vi "Global Strings.vi"() -> ()   [LabVIEW 2024, in "Historical Table.lvlib" / "Historical Table.lvclass"]
uses:
  Historical Table.lvclass
panel:
  in  "Show":string="Show Table"
  in  "Update Period":string="Update period (s)"
  in  "History":string="Hisotry duration (s)"
  in  "Select Channels":string="Select Channels"
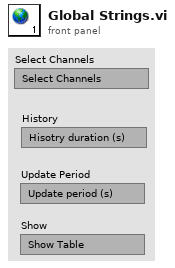
[diagram p1: front panel]
diagram:
